vi "AbbreviateModifications.vi"(4 "svnString":string) -> (1 "VInames":string)   [LabVIEW 2015]
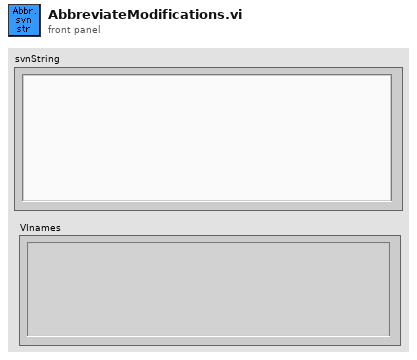
[diagram p1: front panel]
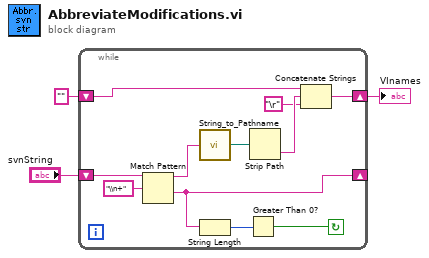
[diagram p0: block diagram]
diagram:
  n1 = while {
    shift-right: [w7] -> _
    shift-left: "svnString" -> [w14]
    shift-right: [w8] -> w1
    shift-left: "" -> [w10]
    stop <- w5 continue-if-true
    n2 = Match Pattern(string=w14, regular expression="\\n+") -> (before substring=w13:string, after substring=w7:string)  [unwired: 1 in, 2 out]
    n3 = call "String_to_Pathname.vi"("Input String"=w13) -> ("path"=w12:path)
    n4 = String Length(string=w7) -> (length=w6:i32)
    n5 = Greater Than 0?(x=w6) -> (x > 0?=w5:bool)
    n6 = Strip Path(path=w12) -> (name=w11:string)  [unwired: 1 out]
    n7 = Concatenate Strings(w10, w11, "\r") -> (w8:string)
  }
  "VInames" <- w1
